vi "Display Custom Shortcut Menu.vi"(8 "error in (no error)":errorcluster, 9 "MenuRef":refnum<k9>, 10 "Ctl Refnum":refnum<vi>, 11 "IControlShortcutMenu In":T1) -> (0 "error out":errorcluster, 2 "Discarded?":bool)   [LabVIEW 2015, in "ActorEvents.lvlib" / "IControlShortcutMenu.lvclass"]
uses:
  IControlShortcutMenu.lvclass
  ControlShortcutMenu Reference.ctl
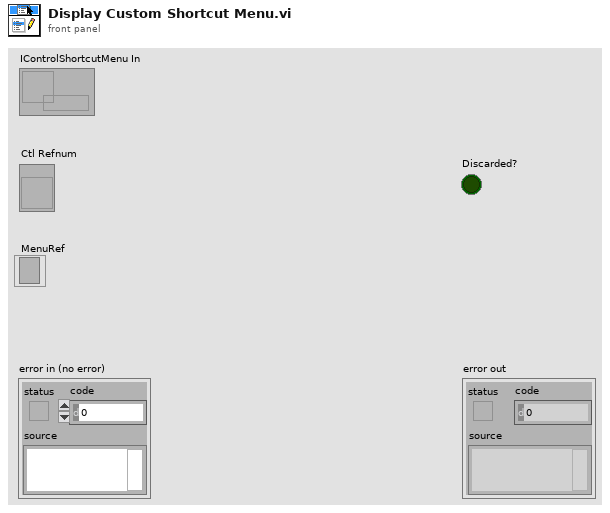
[diagram p1: front panel]
types:
  T1 = typedef "ActorEvents.lvlib/IControlShortcutMenu.lvclass/ControlShortcutMenu Reference.ctl" = refnum<data-value>
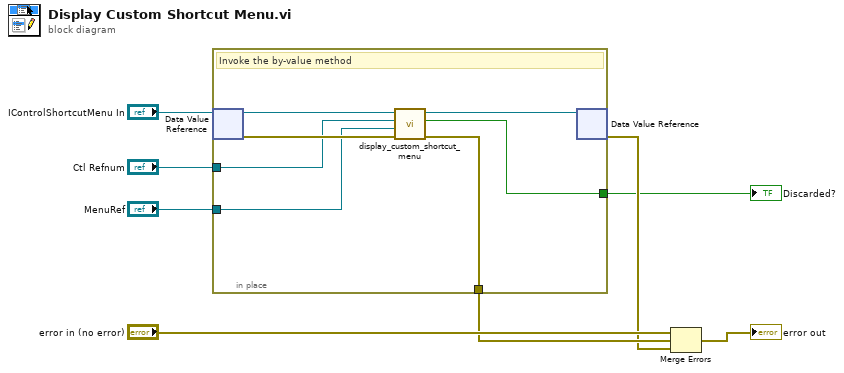
[diagram p0: block diagram]
diagram:
  n1 = in-place {
    in-place-border: "Ctl Refnum" -> [w10]
    in-place-border: "MenuRef" -> [w9]
    in-place-border: [w12] -> w3
    in-place-border: [w11] -> w1
    # "Invoke the by-value method"
    n2 = in-place-dvr #1("IControlShortcutMenu In") -> (w15:refnum<class "IControlShortcutMenu.lvclass">, w13:errorcluster)
    n3 = call-dynamic "display_custom_shortcut_menu.vi"("error in (no error)"=w13, "MenuRef"=w9, "Ctl Refnum"=w10, "IControlShortcutMenu In"=w15) -> ("error out"=w12:errorcluster, "Discarded?"=w11:bool, "IControlShortcutMenu Out"=w14:refnum<class "IControlShortcutMenu.lvclass">)  [unwired: 5 in]
    n4 = in-place-dvr #1(w14) -> (w2:errorcluster)  [unwired: 1 out]
  }
  "Discarded?" <- w1
  n5 = Merge Errors("error in (no error)", w3, w2) -> (→"error out":errorcluster)
